vi "arrayMean.vi"(11 "Array in":dbl[][](array[numeric])) -> (3 "Array out":dbl[](array[numeric]))   [LabVIEW 2014]
doc: "André Romero - 2019\nandretec@ifsc.usp.br"
uses:
  <vilib>/Analysis/baseanly.llb/Mean (DBL).vi
  <vilib>/Analysis/NI_AALBase.lvlib
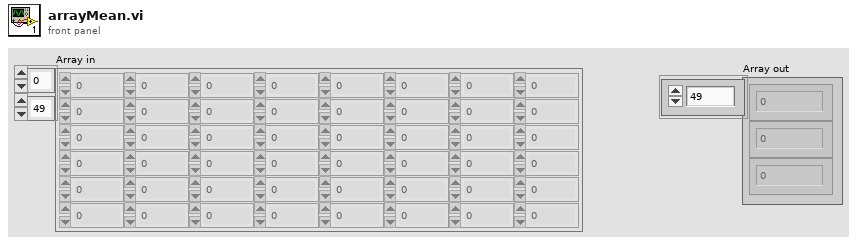
[diagram p1: front panel]
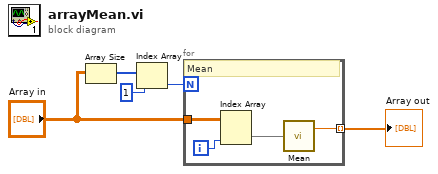
[diagram p0: block diagram]
diagram:
  n1 = Array Size(array="Array in") -> (size(s)=w4:i32[])
  n2 = Index Array(array=w4, index=1) -> (element=w2:i32)
  n3 = for {
    N: w2 -> [_]
    tunnel: "Array in" -> [w9]
    tunnel: [w6] -> w1 mode=indexing
    i -> [w8]
    # "Mean"
    n4 = Index Array(array=w9, index (col)=w8) -> (element=w7:dbl[])  [unwired: 1 in]
    n5 = call-poly <vilib>:"Mean.vi"("X"=w7) -> ("mean"=w6:dbl)  [unwired: 1 out]
  }
  "Array out" <- w1
